vi "HWhist-SimpleImageAcquisition-ScanSyncIn.vi"() -> ()   [LabVIEW 2017]
doc: "This example demonstrates how to use the Becker&Hickl LabVIEW wrapper VIs to acquire one page of data in ScanSyncIn mode. The data is displayed as Sum Of Decays and Intensity Image.\nHere all parameters are hard wired.\nThis VI is based on the C-example part 3 in use_spcm.c\n\ninfo@becker-hickl.com"
uses:
  SPC_Wrappers/SPC_Controls/SPC_RatesCluster.ctl
  SPC_Wrappers/SPC_Controls/StateCluster.ctl
  SPC_Wrappers/SPC_Controls/ConfigMem.ctl
  SPC_Wrappers/SPC_Controls/par_id.ctl
panel:
  out "Clock Status":T1={"Frame Clock"=TRUE, "Line Clock"=TRUE, "Pixel Clock"=TRUE}
  out "SPCMemConfig":T2={"Max Block No"=0, "Blocks Per Frame"=0, "Frames Per Page"=1, "Maxpage"=1, "Block Length"=1} {"Frames Per Page" min=1 step=1; "Maxpage" min=1; "Blocks Per Frame" min=1 step=1}
  out "coltime":sgl(knob) scale=0.0..25.0
  out "SPC_StateCluster":T3
  out "IntensityImage":u32[][](graph)
  in  "Start":bool
  out "SPCRatesCluster":T4={"Sync"=1728.0, "CFD"=1728.0, "TAC"=848.0, "ADC"=144.0} {"Sync" scale=0.0..6000000.0; "ADC" scale=0.0..1000000.0; "TAC" scale=0.0..1000000.0; "CFD" scale=0.0..1000000.0}
  out "SumOfDecays":u32[](graph)=[0, 0, 0, 0, 0, 0, 0, 0, 0, 0, 0, 0, 25, 69, 113, 22834, 49845, 48952, 47008, 44897, 43047, 41676, 39617, 38468, 36759, 35330, 34474, 33046, 31635, 30967, 29469, 28717, 27673, 26421, 26064, 25000, 37648, 768042, 1499623, 1365356, 1091690, 885848, 750159, 647680, 564123, 496756, 447375, 394716, 354643, 325379, 302236, 274792, 253379, 235323, 217869, 201995, 187396, 177487, 163352, 153041, 143962, 135127, 127360, 120248]
  in  "Exit":bool
  out "Serial Number":string[](array[string])
  # "This example demonstrates how to use the Becker&Hickl LabVIEW wrapper VIs to acquire one page of data in ScanSyncIn mode. \nThe data is displayed as Sum Of Decays and Intensity Image.\nHere all parameters are hard wired.                                                                  This VI is based on the C-example part 3 in use_spcm.c"
  # "See Tip-Strip for details"
  # "(c) 2022 Becker & Hickl GmbH\n     ALL RIGHTS RESERVED."
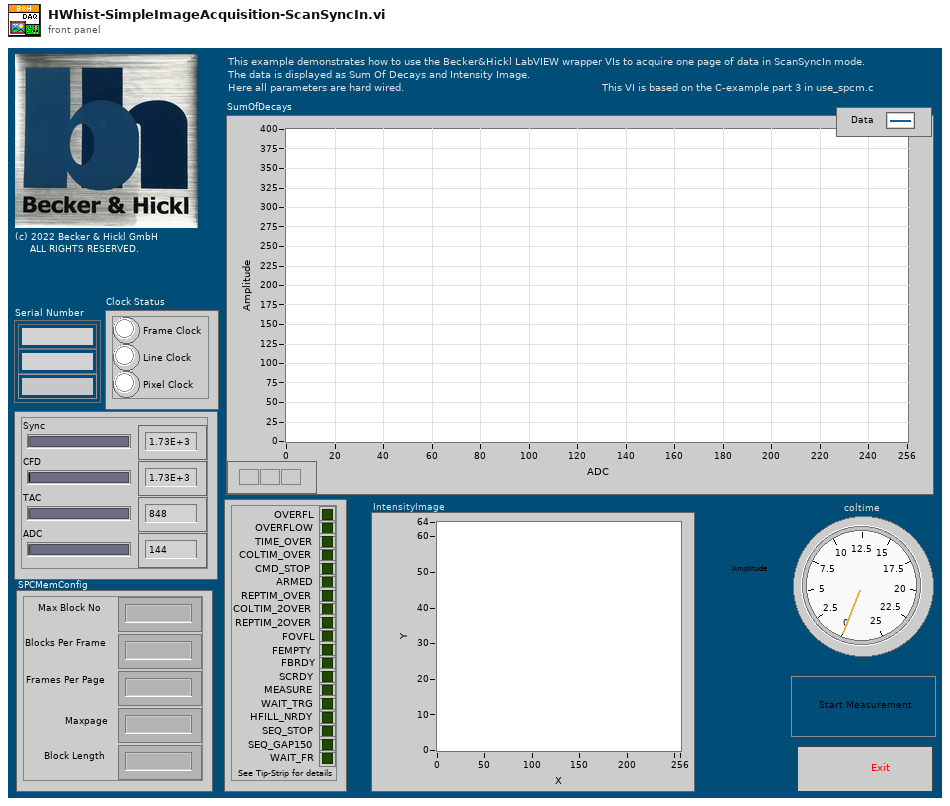
[diagram p1: front panel]
types:
  T1 = cluster{"Frame Clock":bool, "Line Clock":bool, "Pixel Clock":bool}
  T2 = typedef "ConfigMem.ctl" = cluster{"Max Block No":i32, "Blocks Per Frame":i32, "Frames Per Page":i32, "Maxpage":i32, "Block Length":i32}
  T3 = typedef "StateCluster.ctl" = cluster{"OVERFL":bool, "OVERFLOW":bool, "TIME_OVER":bool, "COLTIM_OVER":bool, "CMD_STOP":bool, "ARMED":bool, "REPTIM_OVER":bool, "COLTIM_2OVER":bool, "REPTIM_2OVER":bool, "FOVFL":bool, "FEMPTY":bool, "FBRDY":bool, "SCRDY":bool, "MEASURE":bool, "WAIT_TRG":bool, "HFILL_NRDY":bool, "SEQ_STOP":bool, "SEQ_GAP150":bool, "WAIT_FR":bool}
  T4 = typedef "SPC_RatesCluster.ctl" = cluster{"Sync":sgl, "CFD":sgl, "TAC":sgl, "ADC":sgl}
  T5 = typedef "par_id.ctl" = i16
  T6 = enum16{"IDLE", "Start", "TestState", "Stop", "Read"}
  T7 = typedef "SPCModInfo.ctl" = cluster{"Module Type":T8, "Bus Number":i16, "Slot Number":i16, "in Use":i16, "Init Status":i16, "Base I/O Addr":u16}
  T8 = typedef "ModuleType.ctl" = i16
  T9 = typedef "SPCdata.ctl" = cluster{"base_adr":u16, "init":i16, "cfd_limit_low":sgl, "cfd_limit_high":sgl, "cfd_zc_level":sgl, "cfd_holdoff":sgl, "sync_zc_level":sgl, "sync_holdoff":sgl, "sync_threshold":sgl, "tac_range":sgl, "sync_freq_div":i16, "tac_gain":i16, "tac_offset":sgl, "tac_limit_low":sgl, "tac_limit_high":sgl, "adc_resolution":i16, "ext_latch_delay":i16, "collect_time":sgl, "display_time":sgl, "repeat_time":sgl, "stop_on_time":i16, "stop_on_ovfl":i16, "dither_range":i16, "count_incr":i16, "mem_bank":i16, "dead_time_comp":i16, "scan_control":u16, "routing_mode":u16, "tac_enable_hold":sgl, "pci_card_no":i16, "mode":u16, "scan_size_x":u32, "scan_size_y":u32, "scan_rout_x":u32, "scan_rout_y":u32, "scan_flyback":u32, "scan_borders":u32, "scan_polarity":u16, "pixel_clock":u16, "line_compression":u16, "trigger":u16, "pixel_time":sgl, "ext_pixclk_div":u32, "rate_count_time":sgl, "macro_time_clk":i16, "add_select":i16, "test_eep":i16, "adc_zoom":i16, "img_size_x":u32, "img_size_y":u32, "img_rout_x":u32, "img_rout_y":u32, "xy_gain":i16, "master_clock":i16, "adc_sample_delay":i16, "detector_type":i16, "chan_enable":u32, "chan_slope":u32, "chan_spec_no":u32, "tdc_control":u32, "tdc_offset1":sgl, "tdc_offset2":sgl, "tdc_offset3":sgl, "tdc_offset4":sgl, "future_reserve1":u64, "future_reserve2":u64, "future_reserve3":u64, "future_reserve4":u64, "future_reserve5":u64, "future_reserve6":u64, "future_reserve7":u64}
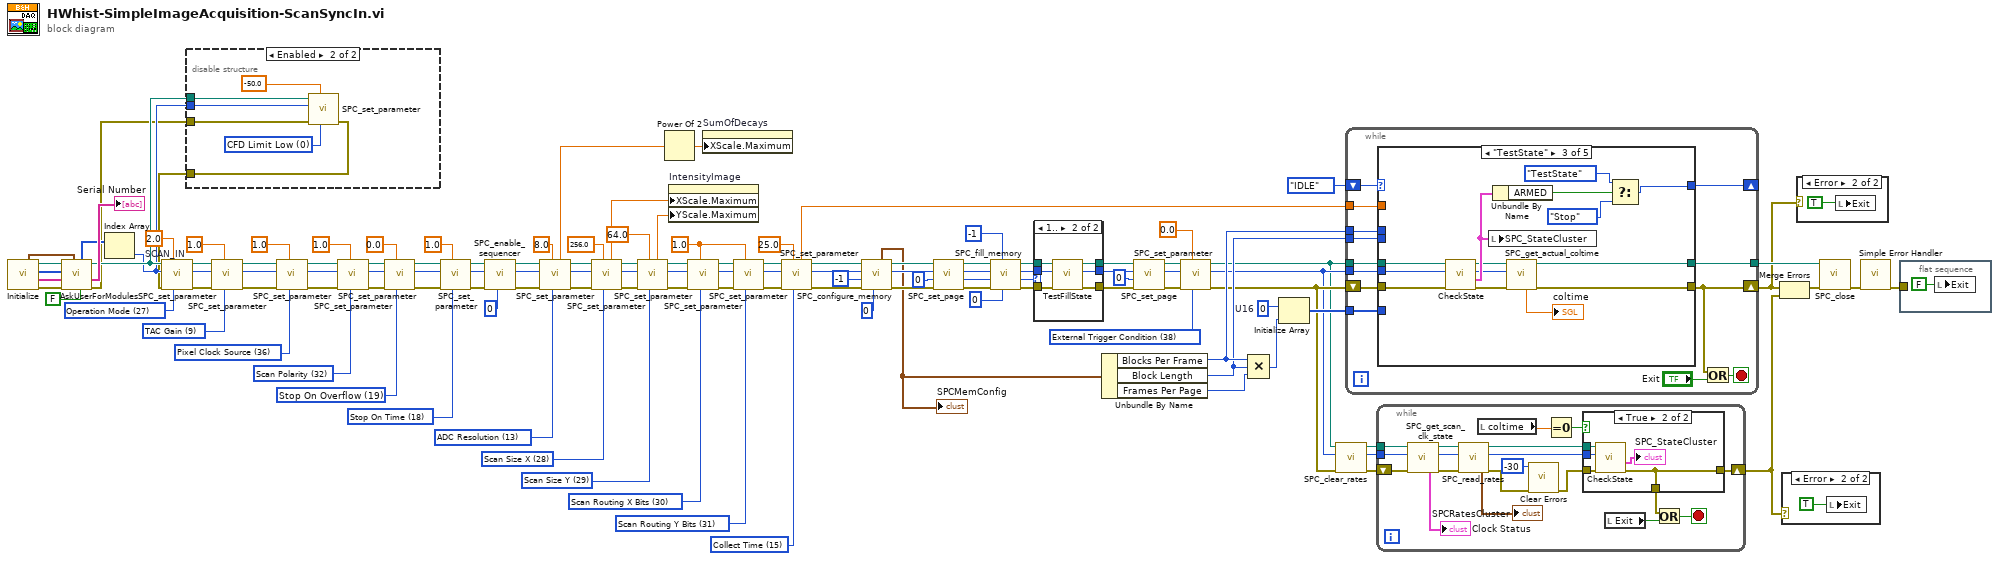
[diagram p0: block diagram]
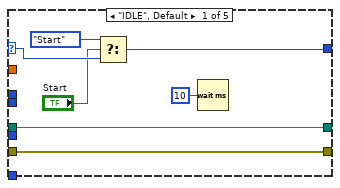
[diagram p2: hidden frame]
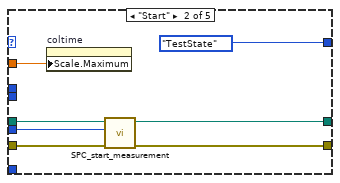
[diagram p3: hidden frame]
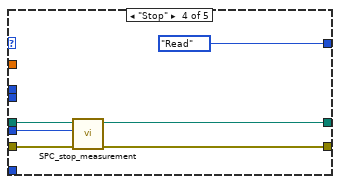
[diagram p4: hidden frame]
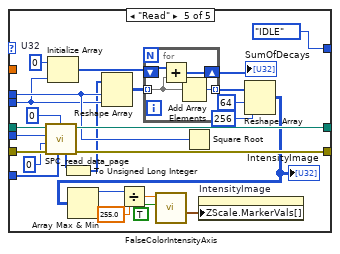
[diagram p5: hidden frame]
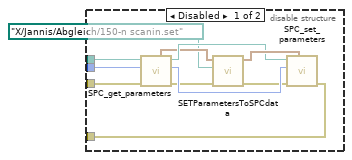
[diagram p9: hidden frame]
diagram:
  w30 = T5 36 items=["CFD Limit Low", "CFD Limit High", "CFD Zero Cross Level", "CFD Holdoff", "SYNC Zero Cross Level", "SYNC Freq Divider", "SYNC Holdoff", "SYNC Threshold", "TAC Range", "TAC Gain", "TAC Offset", "TAC Limit Low", "TAC Limit High", "ADC Resolution", "External Latch Delay", "Collect Time", "Display Time", "Repeat Time", "Stop On Time", "Stop On Overflow", "Dither Range", "Count Increment", "Memory Bank", "Dead Time Compensation", "Scan Control", "Routing Mode", "TAC Enable Hold", "Operation Mode", "Scan Size X", "Scan Size Y", "Scan Routing X Bits", "Scan Routing Y Bits", "Scan Polarity", "Scan Flyback", "Scan Borders", "Pixel Time", "Pixel Clock Source", "Scan Line Compression", "External Trigger Condition", "External Pixel Clock Divider", "Rate Counting Time", "Macro Time Clock", "ADD Signal Source", "ADC Zoom", "XY Gain", "Image Size X", "Image Size Y", "Image Routing X Bits", "Image Routing Y Bits", "Master Clock", "ADC Sample Delay", "Detector Type", "X Axis Type", "Channel Enable", "Channel Slope", "Channel Spec_no"] ("SPC parameter ID")
  w56 = T5 32 items=["CFD Limit Low", "CFD Limit High", "CFD Zero Cross Level", "CFD Holdoff", "SYNC Zero Cross Level", "SYNC Freq Divider", "SYNC Holdoff", "SYNC Threshold", "TAC Range", "TAC Gain", "TAC Offset", "TAC Limit Low", "TAC Limit High", "ADC Resolution", "External Latch Delay", "Collect Time", "Display Time", "Repeat Time", "Stop On Time", "Stop On Overflow", "Dither Range", "Count Increment", "Memory Bank", "Dead Time Compensation", "Scan Control", "Routing Mode", "TAC Enable Hold", "Operation Mode", "Scan Size X", "Scan Size Y", "Scan Routing X Bits", "Scan Routing Y Bits", "Scan Polarity", "Scan Flyback", "Scan Borders", "Pixel Time", "Pixel Clock Source", "Scan Line Compression", "External Trigger Condition", "External Pixel Clock Divider", "Rate Counting Time", "Macro Time Clock", "ADD Signal Source", "ADC Zoom", "XY Gain", "Image Size X", "Image Size Y", "Image Routing X Bits", "Image Routing Y Bits", "Master Clock", "ADC Sample Delay", "Detector Type", "X Axis Type", "Channel Enable", "Channel Slope", "Channel Spec_no"] ("SPC parameter ID")
  w59 = T5 9 items=["CFD Limit Low", "CFD Limit High", "CFD Zero Cross Level", "CFD Holdoff", "SYNC Zero Cross Level", "SYNC Freq Divider", "SYNC Holdoff", "SYNC Threshold", "TAC Range", "TAC Gain", "TAC Offset", "TAC Limit Low", "TAC Limit High", "ADC Resolution", "External Latch Delay", "Collect Time", "Display Time", "Repeat Time", "Stop On Time", "Stop On Overflow", "Dither Range", "Count Increment", "Memory Bank", "Dead Time Compensation", "Scan Control", "Routing Mode", "TAC Enable Hold", "Operation Mode", "Scan Size X", "Scan Size Y", "Scan Routing X Bits", "Scan Routing Y Bits", "Scan Polarity", "Scan Flyback", "Scan Borders", "Pixel Time", "Pixel Clock Source", "Scan Line Compression", "External Trigger Condition", "External Pixel Clock Divider", "Rate Counting Time", "Macro Time Clock", "ADD Signal Source", "ADC Zoom", "XY Gain", "Image Size X", "Image Size Y", "Image Routing X Bits", "Image Routing Y Bits", "Master Clock", "ADC Sample Delay", "Detector Type", "X Axis Type", "Channel Enable", "Channel Slope", "Channel Spec_no"] ("SPC parameter ID")
  w76 = T5 15 items=["CFD Limit Low", "CFD Limit High", "CFD Zero Cross Level", "CFD Holdoff", "SYNC Zero Cross Level", "SYNC Freq Divider", "SYNC Holdoff", "SYNC Threshold", "TAC Range", "TAC Gain", "TAC Offset", "TAC Limit Low", "TAC Limit High", "ADC Resolution", "External Latch Delay", "Collect Time", "Display Time", "Repeat Time", "Stop On Time", "Stop On Overflow", "Dither Range", "Count Increment", "Memory Bank", "Dead Time Compensation", "Scan Control", "Routing Mode", "TAC Enable Hold", "Operation Mode", "Scan Size X", "Scan Size Y", "Scan Routing X Bits", "Scan Routing Y Bits", "Scan Polarity", "Scan Flyback", "Scan Borders", "Pixel Time", "Pixel Clock Source", "Scan Line Compression", "External Trigger Condition", "External Pixel Clock Divider", "Rate Counting Time", "Macro Time Clock", "ADD Signal Source", "ADC Zoom", "XY Gain", "Image Size X", "Image Size Y", "Image Routing X Bits", "Image Routing Y Bits", "Master Clock", "ADC Sample Delay", "Detector Type", "X Axis Type", "Channel Enable", "Channel Slope", "Channel Spec_no"] ("SPC parameter ID")
  w83 = u16 0  # U16
  w87 = T5 38 items=["CFD Limit Low", "CFD Limit High", "CFD Zero Cross Level", "CFD Holdoff", "SYNC Zero Cross Level", "SYNC Freq Divider", "SYNC Holdoff", "SYNC Threshold", "TAC Range", "TAC Gain", "TAC Offset", "TAC Limit Low", "TAC Limit High", "ADC Resolution", "External Latch Delay", "Collect Time", "Display Time", "Repeat Time", "Stop On Time", "Stop On Overflow", "Dither Range", "Count Increment", "Memory Bank", "Dead Time Compensation", "Scan Control", "Routing Mode", "TAC Enable Hold", "Operation Mode", "Scan Size X", "Scan Size Y", "Scan Routing X Bits", "Scan Routing Y Bits", "Scan Polarity", "Scan Flyback", "Scan Borders", "Pixel Time", "Pixel Clock Source", "Scan Line Compression", "External Trigger Condition", "External Pixel Clock Divider", "Rate Counting Time", "Macro Time Clock", "ADD Signal Source", "ADC Zoom", "XY Gain", "Image Size X", "Image Size Y", "Image Routing X Bits", "Image Routing Y Bits", "Master Clock", "ADC Sample Delay", "Detector Type", "X Axis Type", "Channel Enable", "Channel Slope", "Channel Spec_no"] ("SPC parameter ID")
  w99 = sgl 1.0 ("Parameter Value")
  w104 = T5 31 items=["CFD Limit Low", "CFD Limit High", "CFD Zero Cross Level", "CFD Holdoff", "SYNC Zero Cross Level", "SYNC Freq Divider", "SYNC Holdoff", "SYNC Threshold", "TAC Range", "TAC Gain", "TAC Offset", "TAC Limit Low", "TAC Limit High", "ADC Resolution", "External Latch Delay", "Collect Time", "Display Time", "Repeat Time", "Stop On Time", "Stop On Overflow", "Dither Range", "Count Increment", "Memory Bank", "Dead Time Compensation", "Scan Control", "Routing Mode", "TAC Enable Hold", "Operation Mode", "Scan Size X", "Scan Size Y", "Scan Routing X Bits", "Scan Routing Y Bits", "Scan Polarity", "Scan Flyback", "Scan Borders", "Pixel Time", "Pixel Clock Source", "Scan Line Compression", "External Trigger Condition", "External Pixel Clock Divider", "Rate Counting Time", "Macro Time Clock", "ADD Signal Source", "ADC Zoom", "XY Gain", "Image Size X", "Image Size Y", "Image Routing X Bits", "Image Routing Y Bits", "Master Clock", "ADC Sample Delay", "Detector Type", "X Axis Type", "Channel Enable", "Channel Slope", "Channel Spec_no"] ("SPC parameter ID")
  w105 = T5 30 items=["CFD Limit Low", "CFD Limit High", "CFD Zero Cross Level", "CFD Holdoff", "SYNC Zero Cross Level", "SYNC Freq Divider", "SYNC Holdoff", "SYNC Threshold", "TAC Range", "TAC Gain", "TAC Offset", "TAC Limit Low", "TAC Limit High", "ADC Resolution", "External Latch Delay", "Collect Time", "Display Time", "Repeat Time", "Stop On Time", "Stop On Overflow", "Dither Range", "Count Increment", "Memory Bank", "Dead Time Compensation", "Scan Control", "Routing Mode", "TAC Enable Hold", "Operation Mode", "Scan Size X", "Scan Size Y", "Scan Routing X Bits", "Scan Routing Y Bits", "Scan Polarity", "Scan Flyback", "Scan Borders", "Pixel Time", "Pixel Clock Source", "Scan Line Compression", "External Trigger Condition", "External Pixel Clock Divider", "Rate Counting Time", "Macro Time Clock", "ADD Signal Source", "ADC Zoom", "XY Gain", "Image Size X", "Image Size Y", "Image Routing X Bits", "Image Routing Y Bits", "Master Clock", "ADC Sample Delay", "Detector Type", "X Axis Type", "Channel Enable", "Channel Slope", "Channel Spec_no"] ("SPC parameter ID")
  w106 = T5 29 items=["CFD Limit Low", "CFD Limit High", "CFD Zero Cross Level", "CFD Holdoff", "SYNC Zero Cross Level", "SYNC Freq Divider", "SYNC Holdoff", "SYNC Threshold", "TAC Range", "TAC Gain", "TAC Offset", "TAC Limit Low", "TAC Limit High", "ADC Resolution", "External Latch Delay", "Collect Time", "Display Time", "Repeat Time", "Stop On Time", "Stop On Overflow", "Dither Range", "Count Increment", "Memory Bank", "Dead Time Compensation", "Scan Control", "Routing Mode", "TAC Enable Hold", "Operation Mode", "Scan Size X", "Scan Size Y", "Scan Routing X Bits", "Scan Routing Y Bits", "Scan Polarity", "Scan Flyback", "Scan Borders", "Pixel Time", "Pixel Clock Source", "Scan Line Compression", "External Trigger Condition", "External Pixel Clock Divider", "Rate Counting Time", "Macro Time Clock", "ADD Signal Source", "ADC Zoom", "XY Gain", "Image Size X", "Image Size Y", "Image Routing X Bits", "Image Routing Y Bits", "Master Clock", "ADC Sample Delay", "Detector Type", "X Axis Type", "Channel Enable", "Channel Slope", "Channel Spec_no"] ("SPC parameter ID")
  w107 = T5 28 items=["CFD Limit Low", "CFD Limit High", "CFD Zero Cross Level", "CFD Holdoff", "SYNC Zero Cross Level", "SYNC Freq Divider", "SYNC Holdoff", "SYNC Threshold", "TAC Range", "TAC Gain", "TAC Offset", "TAC Limit Low", "TAC Limit High", "ADC Resolution", "External Latch Delay", "Collect Time", "Display Time", "Repeat Time", "Stop On Time", "Stop On Overflow", "Dither Range", "Count Increment", "Memory Bank", "Dead Time Compensation", "Scan Control", "Routing Mode", "TAC Enable Hold", "Operation Mode", "Scan Size X", "Scan Size Y", "Scan Routing X Bits", "Scan Routing Y Bits", "Scan Polarity", "Scan Flyback", "Scan Borders", "Pixel Time", "Pixel Clock Source", "Scan Line Compression", "External Trigger Condition", "External Pixel Clock Divider", "Rate Counting Time", "Macro Time Clock", "ADD Signal Source", "ADC Zoom", "XY Gain", "Image Size X", "Image Size Y", "Image Routing X Bits", "Image Routing Y Bits", "Master Clock", "ADC Sample Delay", "Detector Type", "X Axis Type", "Channel Enable", "Channel Slope", "Channel Spec_no"] ("SPC parameter ID")
  w116 = T5 13 items=["CFD Limit Low", "CFD Limit High", "CFD Zero Cross Level", "CFD Holdoff", "SYNC Zero Cross Level", "SYNC Freq Divider", "SYNC Holdoff", "SYNC Threshold", "TAC Range", "TAC Gain", "TAC Offset", "TAC Limit Low", "TAC Limit High", "ADC Resolution", "External Latch Delay", "Collect Time", "Display Time", "Repeat Time", "Stop On Time", "Stop On Overflow", "Dither Range", "Count Increment", "Memory Bank", "Dead Time Compensation", "Scan Control", "Routing Mode", "TAC Enable Hold", "Operation Mode", "Scan Size X", "Scan Size Y", "Scan Routing X Bits", "Scan Routing Y Bits", "Scan Polarity", "Scan Flyback", "Scan Borders", "Pixel Time", "Pixel Clock Source", "Scan Line Compression", "External Trigger Condition", "External Pixel Clock Divider", "Rate Counting Time", "Macro Time Clock", "ADD Signal Source", "ADC Zoom", "XY Gain", "Image Size X", "Image Size Y", "Image Routing X Bits", "Image Routing Y Bits", "Master Clock", "ADC Sample Delay", "Detector Type", "X Axis Type", "Channel Enable", "Channel Slope", "Channel Spec_no"] ("SPC parameter ID")
  w118 = T5 18 items=["CFD Limit Low", "CFD Limit High", "CFD Zero Cross Level", "CFD Holdoff", "SYNC Zero Cross Level", "SYNC Freq Divider", "SYNC Holdoff", "SYNC Threshold", "TAC Range", "TAC Gain", "TAC Offset", "TAC Limit Low", "TAC Limit High", "ADC Resolution", "External Latch Delay", "Collect Time", "Display Time", "Repeat Time", "Stop On Time", "Stop On Overflow", "Dither Range", "Count Increment", "Memory Bank", "Dead Time Compensation", "Scan Control", "Routing Mode", "TAC Enable Hold", "Operation Mode", "Scan Size X", "Scan Size Y", "Scan Routing X Bits", "Scan Routing Y Bits", "Scan Polarity", "Scan Flyback", "Scan Borders", "Pixel Time", "Pixel Clock Source", "Scan Line Compression", "External Trigger Condition", "External Pixel Clock Divider", "Rate Counting Time", "Macro Time Clock", "ADD Signal Source", "ADC Zoom", "XY Gain", "Image Size X", "Image Size Y", "Image Routing X Bits", "Image Routing Y Bits", "Master Clock", "ADC Sample Delay", "Detector Type", "X Axis Type", "Channel Enable", "Channel Slope", "Channel Spec_no"] ("SPC parameter ID")
  w119 = T5 19 items=["CFD Limit Low", "CFD Limit High", "CFD Zero Cross Level", "CFD Holdoff", "SYNC Zero Cross Level", "SYNC Freq Divider", "SYNC Holdoff", "SYNC Threshold", "TAC Range", "TAC Gain", "TAC Offset", "TAC Limit Low", "TAC Limit High", "ADC Resolution", "External Latch Delay", "Collect Time", "Display Time", "Repeat Time", "Stop On Time", "Stop On Overflow", "Dither Range", "Count Increment", "Memory Bank", "Dead Time Compensation", "Scan Control", "Routing Mode", "TAC Enable Hold", "Operation Mode", "Scan Size X", "Scan Size Y", "Scan Routing X Bits", "Scan Routing Y Bits", "Scan Polarity", "Scan Flyback", "Scan Borders", "Pixel Time", "Pixel Clock Source", "Scan Line Compression", "External Trigger Condition", "External Pixel Clock Divider", "Rate Counting Time", "Macro Time Clock", "ADD Signal Source", "ADC Zoom", "XY Gain", "Image Size X", "Image Size Y", "Image Routing X Bits", "Image Routing Y Bits", "Master Clock", "ADC Sample Delay", "Detector Type", "X Axis Type", "Channel Enable", "Channel Slope", "Channel Spec_no"] ("SPC parameter ID")
  w121 = sgl 2.0  # SCAN_IN
  w122 = T5 27 items=["CFD Limit Low", "CFD Limit High", "CFD Zero Cross Level", "CFD Holdoff", "SYNC Zero Cross Level", "SYNC Freq Divider", "SYNC Holdoff", "SYNC Threshold", "TAC Range", "TAC Gain", "TAC Offset", "TAC Limit Low", "TAC Limit High", "ADC Resolution", "External Latch Delay", "Collect Time", "Display Time", "Repeat Time", "Stop On Time", "Stop On Overflow", "Dither Range", "Count Increment", "Memory Bank", "Dead Time Compensation", "Scan Control", "Routing Mode", "TAC Enable Hold", "Operation Mode", "Scan Size X", "Scan Size Y", "Scan Routing X Bits", "Scan Routing Y Bits", "Scan Polarity", "Scan Flyback", "Scan Borders", "Pixel Time", "Pixel Clock Source", "Scan Line Compression", "External Trigger Condition", "External Pixel Clock Divider", "Rate Counting Time", "Macro Time Clock", "ADD Signal Source", "ADC Zoom", "XY Gain", "Image Size X", "Image Size Y", "Image Routing X Bits", "Image Routing Y Bits", "Master Clock", "ADC Sample Delay", "Detector Type", "X Axis Type", "Channel Enable", "Channel Slope", "Channel Spec_no"] ("SPC parameter ID")
  n1 = call "Initialize.vi"() -> ("ErrorOut"=w124:errorcluster, "SerialNumbersArray"=w80:string[], "ModuleNoArray"=w73:i16[], "DLL Path"=w125:path, "SPCModulesArray"=w65:T7[])  [unwired: 7 in]
  n2 = call "AskUserForModules.vi"("MultiModule"=FALSE, "SPCModulesArray"=w65, "Error In"=w124, "Serial Number"=w80, "ModuleNoArray"=w73, "DLL Path"=w125) -> ("Error Out"=w1:errorcluster, "ActiveSerialNumbers"=→"Serial Number":string[], "DLL Path"=w22:path, "ActiveModuleNo"=w62:i16[])  [unwired: 1 in, 1 out]
  n3 = Index Array(array=w62) -> (element=w21:i16)  [unwired: 1 in]
  n4 = disable-structure shown="Enabled" {
    disable-tunnel: w22 -> [w136 w140]
    disable-tunnel: w21 -> [w135 w139]
    disable-tunnel: [w131 w138] -> w7
    disable-tunnel: w1 -> [w126 w137]
    frame Disabled {
      n5 = call "SPC_get_parameters.vi"("Error In"=w126, "Module No"=w135, "DLL Path"=w136) -> ("Error Out"=w128:errorcluster, "Module No"=w132:i16, "DLL Path"=w133:path, "SPCdata"=w130:T9)  [unwired: 5 in]
      n6 = call "SETParametersToSPCdata.vi"("ErrorIn"=w128, "setFile"=path "X:/Jannis/Abgleich/150-n scanin.set", "SPCdataIn"=w130) -> ("ErrorOut"=w127:errorcluster, "SPCdataOut"=w134:T9)  [unwired: 5 in, 2 out]
      n7 = call "SPC_set_parameters.vi"("SPCdata In"=w134, "Error In"=w127, "Module No."=w132, "DLL Path"=w133) -> ("Error Out"=w131:errorcluster)  [unwired: 4 in, 3 out]
    }
    frame Enabled {
      w142 = T5 0 items=["CFD Limit Low", "CFD Limit High", "CFD Zero Cross Level", "CFD Holdoff", "SYNC Zero Cross Level", "SYNC Freq Divider", "SYNC Holdoff", "SYNC Threshold", "TAC Range", "TAC Gain", "TAC Offset", "TAC Limit Low", "TAC Limit High", "ADC Resolution", "External Latch Delay", "Collect Time", "Display Time", "Repeat Time", "Stop On Time", "Stop On Overflow", "Dither Range", "Count Increment", "Memory Bank", "Dead Time Compensation", "Scan Control", "Routing Mode", "TAC Enable Hold", "Operation Mode", "Scan Size X", "Scan Size Y", "Scan Routing X Bits", "Scan Routing Y Bits", "Scan Polarity", "Scan Flyback", "Scan Borders", "Pixel Time", "Pixel Clock Source", "Scan Line Compression", "External Trigger Condition", "External Pixel Clock Divider", "Rate Counting Time", "Macro Time Clock", "ADD Signal Source", "ADC Zoom", "XY Gain", "Image Size X", "Image Size Y", "Image Routing X Bits", "Image Routing Y Bits", "Master Clock", "ADC Sample Delay", "Detector Type", "X Axis Type", "Channel Enable", "Channel Slope", "Channel Spec_no"] ("SPC parameter ID")
      n8 = call "SPC_set_parameter.vi"("SPC parameter ID"=w142, "Parameter Value"=sgl -50.0, "Error In"=w137, "Module no"=w139, "DLL Path"=w140) -> ("Error Out"=w138:errorcluster)  [unwired: 3 in, 3 out]
    }
  }
  n9 = call "SPC_set_parameter.vi"("SPC parameter ID"=w122, "Parameter Value"=w121, "Error In"=w7, "Module no"=w21, "DLL Path"=w22) -> ("Error Out"=w50:errorcluster, "Module no"=w60:i16, "DLL Path"=w61:path)  [unwired: 3 in, 1 out]
  n10 = call "SPC_set_parameter.vi"("SPC parameter ID"=w59, "Parameter Value"=sgl 1.0, "Error In"=w50, "Module no"=w60, "DLL Path"=w61) -> ("Error Out"=w49:errorcluster, "Module no"=w53:i16, "DLL Path"=w54:path)  [unwired: 3 in, 1 out]
  n11 = call "SPC_set_parameter.vi"("SPC parameter ID"=w30, "Parameter Value"=sgl 1.0, "Error In"=w49, "Module no"=w53, "DLL Path"=w54) -> ("Error Out"=w48:errorcluster, "Module no"=w52:i16, "DLL Path"=w51:path)  [unwired: 3 in, 1 out]
  n12 = call "SPC_set_parameter.vi"("SPC parameter ID"=w56, "Parameter Value"=sgl 1.0, "Error In"=w48, "Module no"=w52, "DLL Path"=w51) -> ("Error Out"=w47:errorcluster, "Module no"=w46:i16, "DLL Path"=w57:path)  [unwired: 3 in, 1 out]
  n13 = call "SPC_set_parameter.vi"("SPC parameter ID"=w119, "Parameter Value"=sgl 0.0, "Error In"=w47, "Module no"=w46, "DLL Path"=w57) -> ("Error Out"=w41:errorcluster, "Module no"=w42:i16, "DLL Path"=w43:path)  [unwired: 3 in, 1 out]
  n14 = call "SPC_set_parameter.vi"("SPC parameter ID"=w118, "Parameter Value"=sgl 1.0, "Error In"=w41, "Module no"=w42, "DLL Path"=w43) -> ("Error Out"=w36:errorcluster, "Module no"=w40:i16, "DLL Path"=w38:path)  [unwired: 3 in, 1 out]
  n15 = call "SPC_enable_sequencer.vi"("Enable"=i16 0, "Error In"=w36, "Module No"=w40, "DLL Path"=w38) -> ("Error Out"=w35:errorcluster, "Module No"=w39:i16, "DLL Path"=w37:path)  [unwired: 5 in]
  n16 = call "SPC_set_parameter.vi"("SPC parameter ID"=w116, "Parameter Value"=sgl 8.0, "Error In"=w35, "Module no"=w39, "DLL Path"=w37) -> ("Error Out"=w108:errorcluster, "Module no"=w109:i16, "DLL Path"=w110:path, "Current Parameter Value"=w2:sgl)  [unwired: 3 in]
  n17 = call "SPC_set_parameter.vi"("SPC parameter ID"=w107, "Parameter Value"=sgl 256.0, "Error In"=w108, "Module no"=w109, "DLL Path"=w110) -> ("Error Out"=w112:errorcluster, "Module no"=w111:i16, "DLL Path"=w100:path, "Current Parameter Value"=w19:sgl)  [unwired: 3 in]
  n18 = call "SPC_set_parameter.vi"("SPC parameter ID"=w106, "Parameter Value"=sgl 64.0, "Error In"=w112, "Module no"=w111, "DLL Path"=w100) -> ("Error Out"=w113:errorcluster, "Module no"=w114:i16, "DLL Path"=w101:path, "Current Parameter Value"=w27:sgl)  [unwired: 3 in]
  n19 = Power Of 2(x=w2) -> (2^x=w3:sgl)
  n20 = property on="IntensityImage" class="IntGraph (strict)"("XScale.Maximum"=w19, "YScale.Maximum"=w27) -> ()  [unwired: 2 in, 2 out]
  n21 = call "SPC_set_parameter.vi"("SPC parameter ID"=w105, "Parameter Value"=w99, "Error In"=w113, "Module no"=w114, "DLL Path"=w101) -> ("Error Out"=w115:errorcluster, "Module no"=w103:i16, "DLL Path"=w102:path)  [unwired: 3 in, 1 out]
  n22 = property on="SumOfDecays" class="WFGraph (strict)"("XScale.Maximum"=w3) -> ()  [unwired: 2 in, 2 out]
  n23 = call "SPC_set_parameter.vi"("SPC parameter ID"=w104, "Parameter Value"=w99, "Error In"=w115, "Module no"=w103, "DLL Path"=w102) -> ("Error Out"=w79:errorcluster, "Module no"=w78:i16, "DLL Path"=w77:path)  [unwired: 3 in, 1 out]
  n24 = call "SPC_set_parameter.vi"("SPC parameter ID"=w76, "Parameter Value"=sgl 25.0, "Error In"=w79, "Module no"=w78, "DLL Path"=w77) -> ("Error Out"=w8:errorcluster, "Module no"=w75:i16, "DLL Path"=w74:path, "Current Parameter Value"=w44:sgl)  [unwired: 3 in]
  n25 = call "SPC_configure_memory.vi"("No of Routing\nChannels"=i16 0 ("Page"), "Error In"=w8, "ADC Resolution [exponent]"=i16 -1 ("Page"), "Module No"=w75, "DLL Path"=w74) -> ("Error Out"=w98:errorcluster, "Module No"=w97:i16, "DLL Path"=w96:path, "SPCMemConfig"=w26:T2)  [unwired: 2 in, 1 out]
  "SPCMemConfig" <- w26
  n26 = call "SPC_set_page.vi"("Error In"=w98, "Page"=0, "Module No"=w97, "DLL Path"=w96) -> ("Error Out"=w93:errorcluster, "Page"=w92:i32, "Module No"=w91:i16, "DLL Path"=w94:path)  [unwired: 4 in]
  n27 = call "SPC_fill_memory.vi"("Fill Value"=u16 0 ("Fill value"), "Block to be Filled"=-1, "Error In"=w93, "Page"=w92, "Module No"=w91, "DLL Path"=w94) -> ("Error Out"=w13:errorcluster, "FunctionReturn"=w14:i16, "Module No"=w15:i16, "DLL Path"=w16:path)  [unwired: 2 in]
  n28 = case shown="1.." w14 {
    tunnel: w16 -> [w144 w151]
    tunnel: w15 -> [w143 w150]
    tunnel: w13 -> [w145 w149]
    tunnel: [w145 w148] -> w11
    tunnel: [w144 w147] -> w10
    tunnel: [w143 w146] -> w9
    frame 0, Default {
    }
    frame 1.. {
      n29 = call "TestFillState.vi"("Error In"=w149, "Module No"=w150, "DLL Path"=w151) -> ("Error Out"=w148:errorcluster, "Module No"=w146:i16, "DLL Path"=w147:path)  [unwired: 6 in]
    }
  }
  n30 = Unbundle By Name(w26) -> ("Blocks Per Frame"=w64:i32, "Block Length"=w63:i32, "Frames Per Page"=w29:i32)
  n31 = call "SPC_set_page.vi"("Error In"=w11, "Page"=0, "Module No"=w9, "DLL Path"=w10) -> ("Error Out"=w31:errorcluster, "Module No"=w32:i16, "DLL Path"=w33:path)  [unwired: 4 in, 1 out]
  n32 = call "SPC_set_parameter.vi"("SPC parameter ID"=w87, "Parameter Value"=sgl 0.0, "Error In"=w31, "Module no"=w32, "DLL Path"=w33) -> ("Error Out"=w6:errorcluster, "Module no"=w5:i16, "DLL Path"=w4:path)  [unwired: 3 in, 1 out]
  n33 = Compound Arithmetic op=MULTIPLY(w64, w63, w29) -> (w66:i32)
  n34 = Initialize Array(w83, w66) -> (w82:u16[])
  n35 = call "SPC_clear_rates.vi"("Error In"=w6, "Module no"=w5, "DLL Path"=w4) -> ("Error Out"=w89:errorcluster, "Module  No"=w88:i16, "DLL Path"=w90:path)  [unwired: 6 in]
  n36 = while {
    shift-right: [w159] -> _
    shift-left: T6."IDLE" -> [w164]
    shift-right: [w156] -> w81
    shift-left: w6 -> [w162]
    tunnel: w5 -> [w160]
    tunnel: w82 -> [w158]
    tunnel: w63 -> [w154]
    tunnel: w64 -> [w153]
    tunnel: w4 -> [w163]
    tunnel: [w161] -> w84
    tunnel: w44 -> [w152]
    stop <- w155 stop-if-true
    n37 = case shown="\"TestState\"" w164 {
      selector: w164 -> [w169 _ _ _ _]
      tunnel: w163 -> [w171 w176 w183 w198 w224]
      tunnel: w162 -> [w170 w178 w189 w197 w223]
      tunnel: [w170 w175 w186 w196 w222] -> w156
      tunnel: [w171 w174 w187 w195 w221] -> w161
      tunnel: w160 -> [_ w177 w182 w194 w220]
      tunnel: [w168 T6."TestState" w191 T6."Read" T6."IDLE"] -> w159
      tunnel: w158 -> [_ _ _ _ w218]
      tunnel: w154 -> [_ _ _ _ w205]
      tunnel: w153 -> [_ _ _ _ w212]
      tunnel: w152 -> [_ w172 _ _ _]
      frame "IDLE", Default {
        n38 = Select(t=T6."Start", s="Start", f=w169) -> (s? t:f=w168:T6)
        n39 = Wait (ms)(milliseconds to wait=u32 10) -> ()  [unwired: 1 out]
      }
      frame "Start" {
        n40 = property on="coltime" class="Knob (strict)"("Scale.Maximum"=w172) -> ()  [unwired: 2 in, 2 out]
        n41 = call "SPC_start_measurement.vi"("Error In"=w178, "Module No"=w177, "DLL Path"=w176) -> ("Error Out"=w175:errorcluster, "DLL Path"=w174:path)  [unwired: 6 in, 1 out]
      }
      frame "TestState" {
        n42 = call "CheckState.vi"("Error In"=w189, "Module No."=w182, "DLL Path"=w183) -> ("Error Out"=w185:errorcluster, "SPC_StateCluster"=w184:T3, "Module No."=w180:i16, "DLL Path"=w181:path)  [unwired: 4 in, 1 out]
        n43 = local write "SPC_StateCluster"(w184) -> ()
        n44 = Unbundle By Name(w184) -> ("ARMED"=w188:bool)
        n45 = call "SPC_get_actual_coltime.vi"("Error In"=w185, "Module No"=w180, "DLL Path"=w181) -> ("Error Out"=w186:errorcluster, "DLL Path"=w187:path, "coltime"=→"coltime":sgl)  [unwired: 5 in, 1 out]
        n46 = Select(t=T6."TestState", s=w188, f=T6."Stop") -> (s? t:f=w191:T6)
      }
      frame "Stop" {
        n47 = call "SPC_stop_measurement.vi"("Error In"=w197, "Module No"=w194, "DLL Path"=w198) -> ("Error Out"=w196:errorcluster, "DLL Path"=w195:path)  [unwired: 6 in, 1 out]
      }
      frame "Read" {
        w215 = u32 0  # U32
        n48 = call "SPC_read_data_page.vi"("DataBuffer"=w218, "First Page"=0, "Error In"=w223, "Last Page"=0, "Module No"=w220, "DLL Path"=w224) -> ("Error Out"=w222:errorcluster, "DLL Path"=w221:path, "Output Data"=w204:u16[])  [unwired: 2 in, 1 out]
        n49 = Initialize Array(w215, w205) -> (w214:u32[])
        n50 = To Unsigned Long Integer(number=w204) -> (unsigned 32bit integer=w203:u32[])
        n51 = Reshape Array(w203, w212, w205) -> (w202:u32[][])
        n52 = for {
          tunnel: w202 -> [w225] mode=indexing
          tunnel: [w228] -> w199 mode=indexing
          shift-right: [w226] -> w213
          shift-left: w214 -> [w227]
          n53 = Add(x=w227, y=w225) -> (x+y=w226:u32[])
          n54 = Add Array Elements(numeric array=w225) -> (sum=w228:u32)
        }
        "SumOfDecays" <- w213
        n55 = Square Root(x=w212) -> ()  [unwired: 1 out]
        n56 = Reshape Array(w199, 64 ("dimension size"), 256 ("dimension size")) -> (w206:u32[][])
        "IntensityImage" <- w206
        n57 = Array Max & Min(array=w206) -> (max value=w211:u32)  [unwired: 3 out]
        n58 = Divide(x=w211, y=255.0) -> (x/y=w208:dbl)
        n59 = call "FalseColorIntensityAxis.vi"("ViewColor"=TRUE, "Scale"=w208) -> ("ZScaleMarkerVals"=w210:cluster{dbl, "Color Box":u32}[])  [unwired: 9 in]
        n60 = property on="IntensityImage" class="IntGraph (strict)"("ZScale.MarkerVals[]"=w210) -> ()  [unwired: 2 in, 2 out]
      }
    }
    n61 = Or(x=w156, y="Exit") -> (x .or. y?=w155:bool)
  }
  n62 = while {
    tunnel: w88 -> [w233]
    shift-right: [w236] -> w71
    shift-left: w89 -> [w235]
    tunnel: w90 -> [w232]
    stop <- w244 stop-if-true
    n63 = call "SPC_get_scan_clk_state.vi"("Error In"=w235, "Module No"=w233, "DLL Path"=w232) -> ("Error Out"=w234:errorcluster, "Module No"=w230:i16, "DLL Path"=w231:path, "Clock Status"=→"Clock Status":T1)  [unwired: 4 in, 1 out]
    n64 = call "SPC_read_rates.vi"("Error In"=w234, "Module No"=w230, "DLL Path"=w231) -> ("Error Out"=w247:errorcluster, "Module No"=w239:i16, "DLL Path"=w240:path, "SPC_RatesCluster"=→"SPCRatesCluster":T4)  [unwired: 5 in]
    n65 = local read "coltime"() -> (w238:sgl)
    n66 = call <vilib>:"Clear Errors.vi"("error in (no error)"=w247, "specific error code to clear (0: all)"=-30) -> ("error out"=w242:errorcluster)  [unwired: 4 in, 1 out]
    n67 = Equal To 0?(x=w238) -> (x = 0?=w237:bool)
    n68 = case shown="True" w237 {
      tunnel: w242 -> [w248 w253]
      tunnel: [w248 w249] -> w241
      tunnel: w240 -> [_ w252]
      tunnel: w239 -> [_ w251]
      tunnel: [w248 w249] -> w236
      frame False {
      }
      frame True {
        n69 = call "CheckState.vi"("Error In"=w253, "Module No."=w251, "DLL Path"=w252) -> ("Error Out"=w249:errorcluster, "SPC_StateCluster"=→"SPC_StateCluster":T3)  [unwired: 4 in, 3 out]
      }
    }
    n70 = local read "Exit"() -> (w245:bool)
    n71 = Or(x=w241, y=w245) -> (x .or. y?=w244:bool)
  }
  n72 = Merge Errors(w81, w71) -> (w72:errorcluster)
  n73 = case shown="Error" w71 {
    frame No Error {
    }
    frame Error {
      n74 = local write "Exit"(TRUE) -> ()
    }
  }
  n75 = case shown="Error" w81 {
    frame No Error {
    }
    frame Error {
      n76 = local write "Exit"(TRUE) -> ()
    }
  }
  n77 = call "SPC_close.vi"("Error In"=w72, "DLL Path"=w84) -> ("Error Out"=w70:errorcluster)  [unwired: 8 in, 1 out]
  n78 = call <vilib>:"Simple Error Handler.vi"("error in (no error)"=w70) -> ("error out"=w69:errorcluster)  [unwired: 4 in, 4 out]
  n79 = flat-sequence {
    tunnel: w69 -> [_]
    frame #0 {
      n80 = local write "Exit"(FALSE) -> ()
    }
  }
